vi "Kick Problem Fix.vi"(1 "Kick Info Modified":T1, 2 "Kick Info Original":T1) -> (0 "Kick Info Fixed":T1)   [LabVIEW 2013]
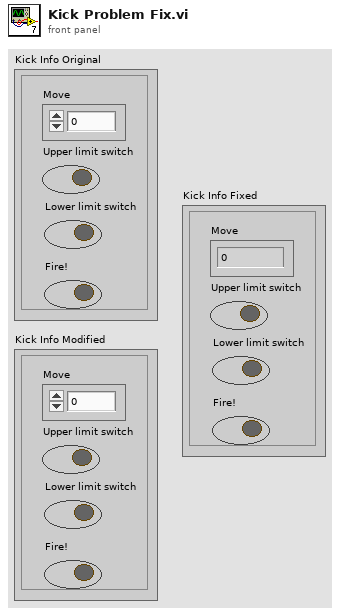
[diagram p1: front panel]
types:
  T1 = cluster{"Move":dbl, "Upper limit switch":bool, "Lower limit switch ":bool, "Fire!":bool}
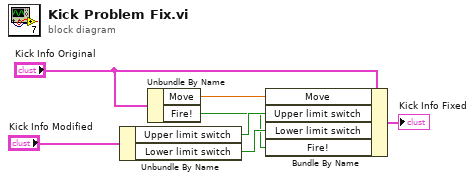
[diagram p0: block diagram]
diagram:
  n1 = Unbundle By Name("Kick Info Modified") -> ("Upper limit switch"=w7:bool, "Lower limit switch"=w6:bool)
  n2 = Unbundle By Name("Kick Info Original") -> ("Move"=w5:dbl, "Fire!"=w3:bool)
  n3 = Bundle By Name(cluster="Kick Info Original", "Move"=w5, "Upper limit switch"=w7, "Lower limit switch"=w6, "Fire!"=w3) -> (→"Kick Info Fixed":T1)
